vi "teststreamer server.vi"() -> ()   [LabVIEW 2016]
uses:
  dllwrapper/action complete event.ctl
  tls classes/connection creator/server acceptor/server acceptor.lvclass
  C:/Users/IEUser/Desktop/libasynclvtls/tls classes/connection creator/connection creator.lvclass
  tls classes/connection/connection.lvclass
  tls classes/engine context/engine context.lvclass
  tls classes/connection creator/connection creator.lvclass
  dllwrapper/async tls dl.lvlib
  <vilib>/ptbypt/NI_PtbyPt.lvlib
panel:
  in  "dimension size":i32=50000
  out "Numeric":dbl
  out "Waveform Chart":dbl(graph)
  out "bytes/s":dbl
  out "bytes written":i32
  in  "stop":bool
  out "error out 3":errorcluster
  out "error out 2":errorcluster
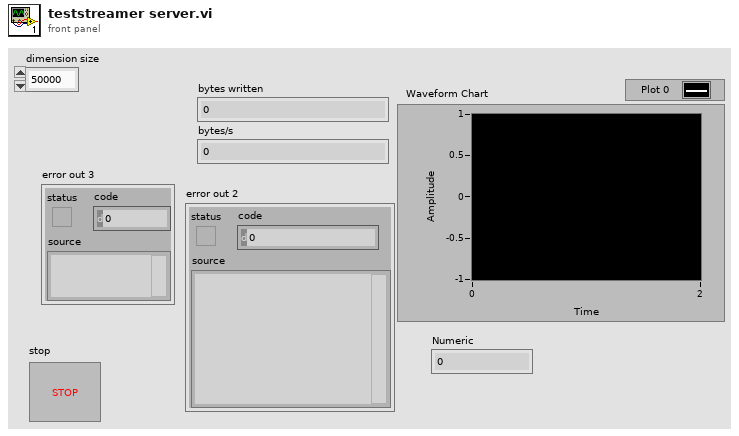
[diagram p1: front panel]
types:
  T1 = typedef "async tls dl.lvlib/action complete event.ctl" = cluster{"request ID":u32, "error code":i32, "error string":string}
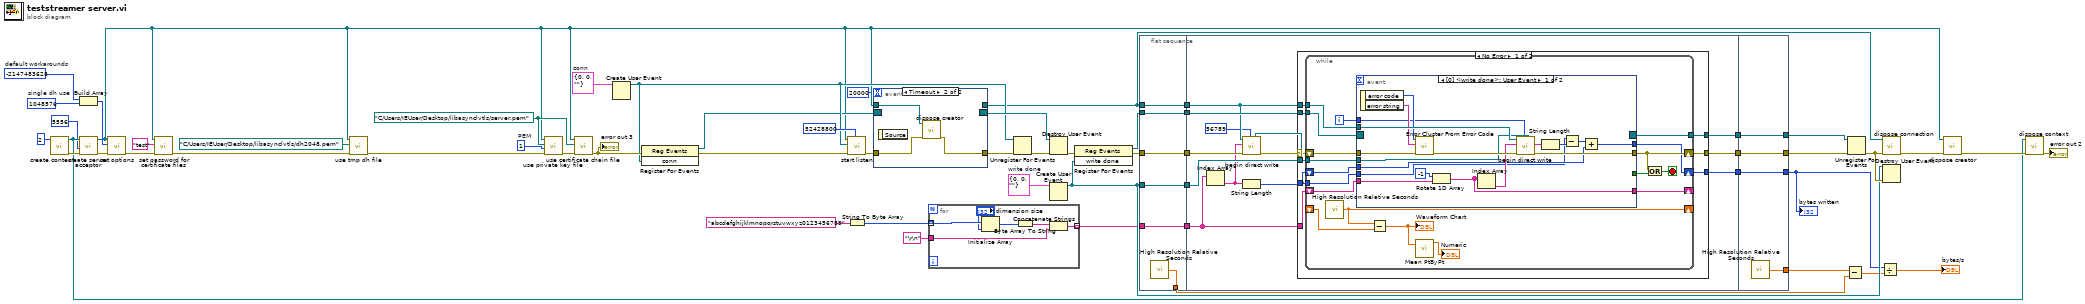
[diagram p0: block diagram]
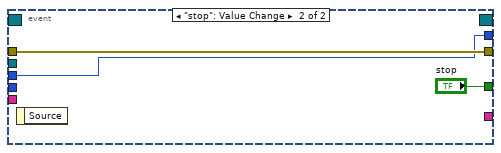
[diagram p2: hidden frame]
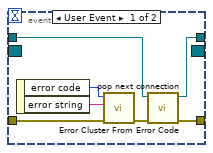
[diagram p4: hidden frame]
diagram:
  w28 = T1 {"request ID"=0, "error code"=0, "error string"=""}  # write done
  w38 = T1 {"request ID"=0, "error code"=0, "error string"=""}  # conn
  w43 = 1  # PEM
  w48 = path "C:/Users/IEUser/Desktop/libasynclvtls/server.pem" ("cert chain file")
  w51 = -2147483628  # default workarounds
  w52 = 1048576  # single dh use
  n1 = call "create context.vi"("thread count"=u64 2) -> ("error out"=w55:errorcluster, "engine context out"=w54:refnum<class "engine context.lvclass">)  [unwired: 9 in]
  n2 = Build Array(w51, w52) -> (w45:i32[])
  n3 = call "create server acceptor.vi"("error in"=w55, "port"=u16 5556, "engine context in"=w54) -> ("error out"=w53:errorcluster, "server acceptor out"=w23:refnum<class "server acceptor.lvclass">)  [unwired: 7 in]
  n4 = call "set options.vi"("error in"=w53, "options"=w45, "connection creator in"=w23) -> ("error out"=w50:errorcluster)  [unwired: 8 in]
  n5 = call "set password for certificate files.vi"("error in"=w50, "password"="test" ("file"), "connection creator in"=w23) -> ("error out"=w42:errorcluster)  [unwired: 8 in]
  n6 = call "use tmp dh file.vi"("error in"=w42, "tmp dh file"=path "C:/Users/IEUser/Desktop/libasynclvtls/dh2048.pem", "connection creator in"=w23) -> ("error out"=w41:errorcluster)  [unwired: 8 in]
  n7 = call "use private key file.vi"("error in"=w41, "format"=w43, "private key file"=w48, "connection creator in"=w23) -> ("error out"=w40:errorcluster)  [unwired: 7 in]
  n8 = call "use certificate chain file.vi"("error in"=w40, "cert chain file"=w48, "connection creator in"=w23) -> ("error out"=w47:errorcluster)  [unwired: 8 in]
  "error out 3" <- w47
  n9 = Create User Event(user event datatype=w38) -> (user event=w33:refnum<user-event>)  [unwired: 1 in, 1 out]
  n10 = register-events(error in=w47, w33) -> (reference out=w29:refnum<event-registration>, error out=w37:errorcluster)  [unwired: 1 in]
  n11 = call "start listen.vi"("stream buffer size"=u64 52428800, "error in"=w37, "completion event"=w33, "server acceptor in"=w23) -> ("error out"=w31:errorcluster)  [unwired: 7 in]
  n12 = String To Byte Array(string="abcdefghijklmnopqrstuvwxyz0123456789") -> (unsigned byte array=w21:u8[])
  n13 = event shown="[1] Timeout" {
    selector: w29 -> [_ _]
    dyn-events: [_ _] -> w30
    timeout: 20000 -> [_ _]
    tunnel: [w63 w66] -> w32
    tunnel: w31 -> [w64 w67]
    tunnel: w23 -> [w59 w65]
    tunnel: [w58 _] -> w22
    event User Event {
      n14 = event-data() -> ("error code"=w61:i32, "error string"=w60:string)  [unwired: 1 in]
      n15 = call <vilib>:"Error Cluster From Error Code.vi"("error in (no error)"=w64, "error message (\"\")"=w60, "error code (0)"=w61) -> ("error out"=w62:errorcluster)  [unwired: 6 in]
      n16 = call "pop next connection.vi"("error in"=w62, "connection creator in"=w59) -> ("error out"=w63:errorcluster, "connection out"=w58:refnum<class "connection.lvclass">)  [unwired: 8 in]
    }
    event Timeout {
      n17 = event-data() -> ()  [unwired: 1 in, 1 out]
      n18 = call "dispose creator.vi"("error in"=w67, "connection creator in"=w65) -> ("error out"=w66:errorcluster)  [unwired: 9 in]
    }
  }
  n19 = for {
    tunnel: w21 -> [w73] mode=indexing
    tunnel: [w70] -> w17 mode=indexing
    tunnel: "\r\n" ("termination") -> [w69]
    n20 = Initialize Array(w73, "dimension size") -> (w72:u8[])
    n21 = Byte Array To String(unsigned byte array=w72) -> (string=w71:string)
    n22 = Concatenate Strings(w71, w69) -> (w70:string)
  }
  n23 = Unregister For Events(event registration refnum=w30, error in=w32) -> (error out=w36:errorcluster)
  n24 = Destroy User Event(user event=w33, error in=w36) -> (error out=w35:errorcluster)
  n25 = Create User Event(user event datatype=w28) -> (user event=w18:refnum<user-event>)  [unwired: 1 in, 1 out]
  n26 = register-events(error in=w35, w18) -> (reference out=w27:refnum<event-registration>, error out=w34:errorcluster)  [unwired: 1 in]
  n27 = flat-sequence {
    tunnel: w17 -> [w75]
    tunnel: w18 -> [w76]
    tunnel: w22 -> [w77]
    tunnel: w27 -> [w78]
    tunnel: w34 -> [w79]
    tunnel: [w79] -> w16
    tunnel: [w78] -> w15
    tunnel: [w77] -> w14
    tunnel: [w76] -> w13
    tunnel: [w75] -> w12
    tunnel: [w74] -> w8
    tunnel: w16 -> [w91]
    tunnel: w15 -> [w90]
    tunnel: w14 -> [w87]
    tunnel: w13 -> [w86]
    tunnel: w12 -> [w85]
    tunnel: [w89] -> w11
    tunnel: [w88] -> w10
    tunnel: [w84] -> w7
    tunnel: [w144] -> w24
    tunnel: [w145] -> w26
    tunnel: w11 -> [w145]
    tunnel: w10 -> [w144]
    tunnel: [w143] -> w9
    tunnel: [w142] -> w5
    tunnel: w7 -> [w142]
    frame #0 {
      n28 = call <vilib>:"High Resolution Relative Seconds.vi"() -> ("relative seconds"=w74:dbl)
    }
    frame #1 {
      n29 = Index Array(array=w85) -> (element=w81:string)  [unwired: 1 in]
      n30 = call "begin direct write.vi"("event"=w86, "id"=u32 56789, "error in"=w91, "data"=w81, "connection in"=w87) -> ("error out"=w82:errorcluster)  [unwired: 5 in, 1 out]
      n31 = String Length(string=w81) -> (length=w80:i32)
      n32 = case shown="No Error" w82 {
        selector: w82 -> [w93 w140]
        tunnel: w90 -> [w100 w141]
        tunnel: [w99 w140] -> w89
        tunnel: [w98 w141] -> w88
        tunnel: w87 -> [w97 _]
        tunnel: w86 -> [w96 _]
        tunnel: w85 -> [w95 _]
        tunnel: [w94 _] -> w84
        tunnel: w80 -> [w92 _]
        frame No Error {
          n33 = while {
            tunnel: w100 -> [w118]
            shift-right: [w114] -> w99
            shift-left: w93 -> [w117]
            tunnel: w97 -> [w116]
            tunnel: [w112] -> w98
            tunnel: w96 -> [w111]
            shift-right: [w109] -> _
            shift-left: w95 -> [w110]
            tunnel: w92 -> [w107]
            shift-right: [w106] -> w94
            shift-left: w92 -> [w105]
            shift-right: [w103] -> _
            shift-left: _ -> [w104]
            i -> [w108]
            stop <- w115 stop-if-true
            n34 = call <vilib>:"High Resolution Relative Seconds.vi"() -> ("relative seconds"=w103:dbl)
            n35 = event shown="[0] <write done>: User Event" {
              selector: w118 -> [_ _]
              dyn-events: [_ _] -> w112
              timeout: _ -> [_ _]
              tunnel: w117 -> [w136 w138]
              tunnel: w116 -> [w134 _]
              tunnel: [w135 w138] -> w114
              tunnel: [_ "stop"] -> w113
              tunnel: w111 -> [w129 _]
              tunnel: w110 -> [w130 _]
              tunnel: [w126 _] -> w109
              tunnel: w108 -> [w128 _]
              tunnel: w107 -> [w120 _]
              tunnel: [w123 w137] -> w106
              tunnel: w105 -> [w122 w137]
              event User Event {
                n36 = event-data() -> ("error code"=w131:i32, "error string"=w132:string)  [unwired: 1 in]
                n37 = call <vilib>:"Error Cluster From Error Code.vi"("error in (no error)"=w136, "error message (\"\")"=w132, "error code (0)"=w131) -> ("error out"=w133:errorcluster)  [unwired: 6 in]
                n38 = Rotate 1D Array(1:w130, 2:-1 ("n")) -> (0:w126:string[])
                n39 = Index Array(array=w126) -> (element=w125:string)  [unwired: 1 in]
                n40 = call "begin direct write.vi"("event"=w129, "id"=w128, "error in"=w133, "data"=w125, "connection in"=w134) -> ("error out"=w135:errorcluster, "remaining data"=w124:string)  [unwired: 5 in]
                n41 = String Length(string=w124) -> (length=w121:i32)
                n42 = Subtract(x=w120, y=w121) -> (x-y=w119:i32)
                n43 = Add(x=w119, y=w122) -> (x+y=w123:i32)
              }
              event "stop": Value Change {
                n44 = event-data() -> ()  [unwired: 1 in, 1 out]
              }
            }
            n45 = Subtract(x=w103, y=w104) -> (x-y=w101:dbl)
            "Waveform Chart" <- w101
            n46 = call <vilib>:"Mean PtByPt.vi"("x"=w101) -> ("mean"=→"Numeric":dbl)  [unwired: 3 in, 1 out]
            n47 = Or(x=w114, y=w113) -> (x .or. y?=w115:bool)
          }
        }
        frame Error {
        }
      }
    }
    frame #2 {
      n48 = call <vilib>:"High Resolution Relative Seconds.vi"() -> ("relative seconds"=w143:dbl)
    }
  }
  n49 = Subtract(x=w9, y=w8) -> (x-y=w6:dbl)
  n50 = Unregister For Events(event registration refnum=w24, error in=w26) -> (error out=w25:errorcluster)
  n51 = Divide(x=w5, y=w6) -> (x/y=→"bytes/s":dbl)
  n52 = call "dispose connection.vi"("error in"=w25, "connection in"=w22) -> ("error out"=w57:errorcluster)  [unwired: 9 in]
  n53 = Destroy User Event(user event=w18, error in=w25) -> ()  [unwired: 1 out]
  n54 = call "dispose creator.vi"("error in"=w57, "connection creator in"=w23) -> ("error out"=w56:errorcluster)  [unwired: 9 in]
  n55 = call "dispose context.vi"("error in"=w56, "engine context out"=w54) -> ("error out"=→"error out 2":errorcluster)  [unwired: 9 in]
  "bytes written" <- w5
